vi "Generate skewed triangular waveform.vi"(4 "Duty cycle (%)":dbl, 5 "Offset":dbl, 6 "sampling info":cluster{"Fs":dbl, "#s":dbl}={"Fs"=1000.0, "#s"=1000.0} {"Fs" format="%.2p"}, 8 "error in (no error)":errorcluster, 9 "Phase":dbl, 10 "Amplitude":dbl, 11 "Frequency":dbl) -> (0 "error out":errorcluster, 3 "Waveform":waveform(dbl))   [LabVIEW 2012]
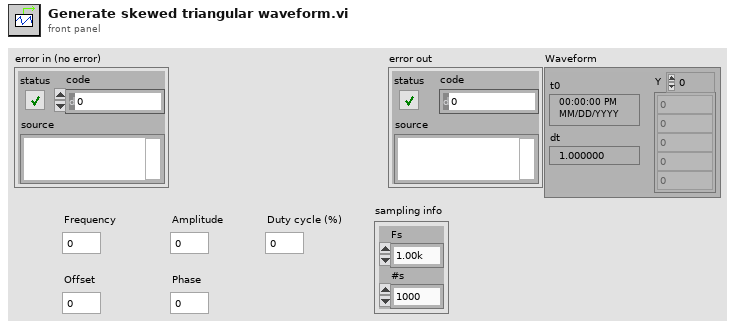
[diagram p1: front panel]
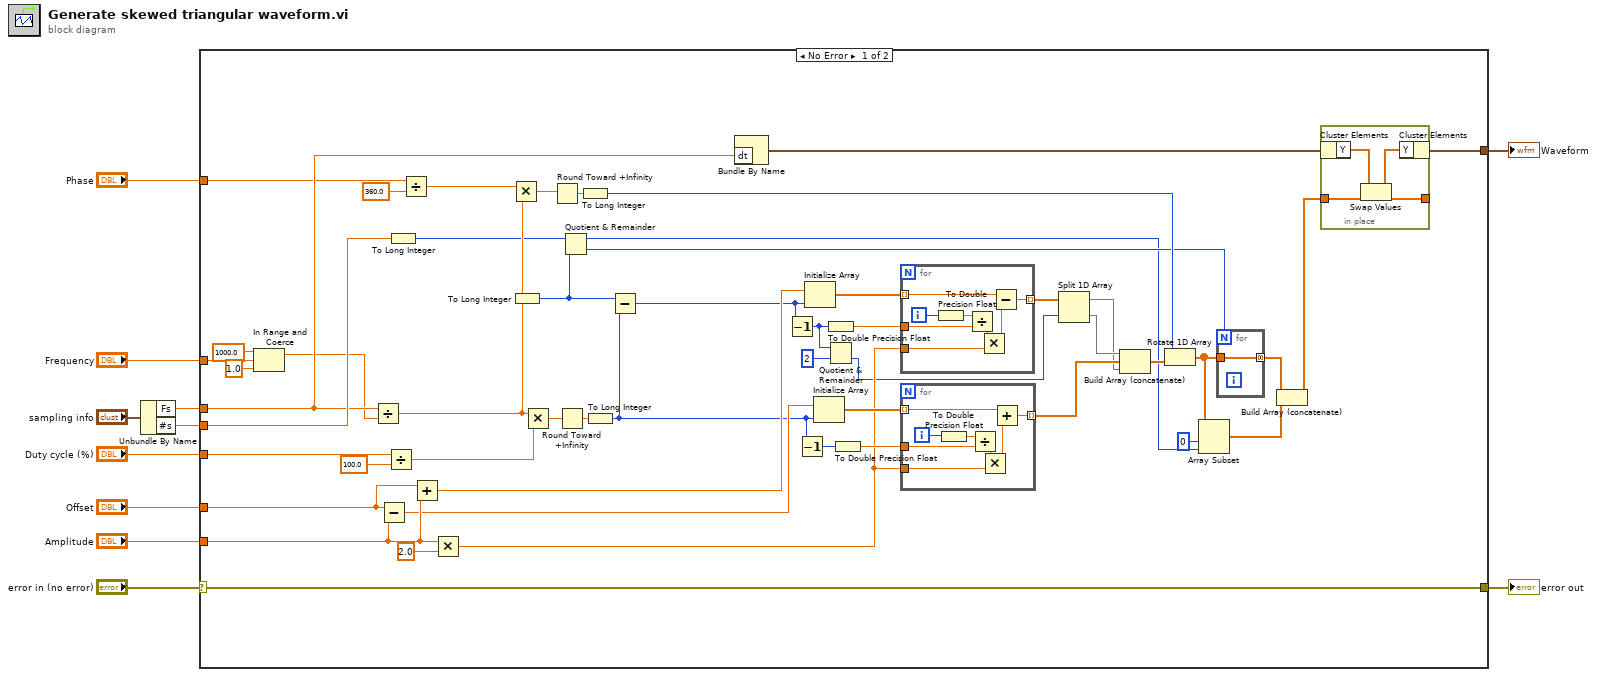
[diagram p0: block diagram]
diagram:
  n1 = Unbundle By Name("sampling info") -> ("Fs"=w4:dbl, "#s"=w7:dbl)
  n2 = case shown="No Error" "error in (no error)" {
    selector: "error in (no error)" -> [w56 w84]
    tunnel: [w56 w84] -> w10
    tunnel: [w55 _] -> w9
    tunnel: w7 -> [w62 _]
    tunnel: "Duty cycle (%)" -> [w61 _]
    tunnel: "Frequency" -> [w13 _]
    tunnel: w4 -> [w60 _]
    tunnel: "Amplitude" -> [w59 _]
    tunnel: "Offset" -> [w58 _]
    tunnel: "Phase" -> [w57 _]
    frame No Error {
      n3 = In Range and Coerce(upper limit=1000.0, x=w13, lower limit=1.0) -> (coerced(x)=w12:dbl)  [unwired: 1 out]
      n4 = Divide(x=w60, y=w12) -> (x/y=w32:dbl)
      n5 = Subtract(x=w58, y=w59) -> (x-y=w47:dbl)
      n6 = Divide(x=w61, y=100.0) -> (x/y=w53:dbl)
      n7 = To Long Integer(number=w62) -> (32bit integer=w29:i32)
      n8 = Divide(x=w57, y=360.0) -> (x/y=w31:dbl)
      n9 = Add(x=w58, y=w59) -> (x+y=w46:dbl)
      n10 = Multiply(x=w59, y=2.0) -> (x*y=w39:dbl)
      n11 = Multiply(x=w31, y=w32) -> (x*y=w35:dbl)
      n12 = To Long Integer(number=w32) -> (32bit integer=w30:i32)
      n13 = Multiply(x=w32, y=w53) -> (x*y=w50:dbl)
      n14 = Round Toward +Infinity(x=w35) -> (ceil(x): smallest int >= x=w36:dbl)
      n15 = Round Toward +Infinity(x=w50) -> (ceil(x): smallest int >= x=w54:dbl)
      n16 = Quotient & Remainder(x=w29, y=w30) -> (x-y*floor(x/y)=w26:i32, floor(x/y)=w28:i32)
      n17 = To Long Integer(number=w36) -> (32bit integer=w33:i32)
      n18 = To Long Integer(number=w54) -> (32bit integer=w45:i32)
      n19 = Subtract(x=w30, y=w45) -> (x-y=w43:i32)
      n20 = Bundle By Name("dt"=w60) -> (w51:waveform(dbl))  [unwired: 1 in]
      n21 = Decrement(x=w43) -> (x-1=w20:i32)
      n22 = Decrement(x=w45) -> (x-1=w42:i32)
      n23 = Initialize Array(w46, w43) -> (w48:dbl[])
      n24 = Initialize Array(w47, w45) -> (w49:dbl[])
      n25 = To Double Precision Float(number=w20) -> (double precision float=w40:dbl)
      n26 = Quotient & Remainder(x=w20, y=2) -> (floor(x/y)=w18:i32)  [unwired: 1 out]
      n27 = To Double Precision Float(number=w42) -> (double precision float=w41:dbl)
      n28 = for {
        tunnel: w48 -> [w65] mode=indexing
        tunnel: w40 -> [w69]
        tunnel: w39 -> [w68]
        tunnel: [w64] -> w21 mode=indexing
        i -> [w71]
        n29 = To Double Precision Float(number=w71) -> (double precision float=w70:dbl)
        n30 = Divide(x=w70, y=w69) -> (x/y=w67:dbl)
        n31 = Multiply(x=w67, y=w68) -> (x*y=w66:dbl)
        n32 = Subtract(x=w65, y=w66) -> (x-y=w64:dbl)
      }
      n33 = for {
        tunnel: w49 -> [w74] mode=indexing
        tunnel: w41 -> [w77]
        tunnel: w39 -> [w75]
        tunnel: [w72] -> w38 mode=indexing
        i -> [w79]
        n34 = To Double Precision Float(number=w79) -> (double precision float=w78:dbl)
        n35 = Divide(x=w78, y=w77) -> (x/y=w76:dbl)
        n36 = Multiply(x=w76, y=w75) -> (x*y=w73:dbl)
        n37 = Add(x=w74, y=w73) -> (x+y=w72:dbl)
      }
      n38 = Split 1D Array(array=w21, index=w18) -> (first subarray=w16:dbl[], second subarray=w17:dbl[])
      n39 = Build Array (concatenate)(w17, w38, w16) -> (w34:dbl[])
      n40 = Rotate 1D Array(1:w34, 2:w33) -> (0:w27:dbl[])
      n41 = Array Subset(array=w27, index=0, length=w26) -> (w24:dbl[])
      n42 = for {
        N: w28 -> [_]
        tunnel: w27 -> [w63]
        tunnel: [w63] -> w23 mode=concatenating
      }
      n43 = Build Array (concatenate)(w23, w24) -> (w22:dbl[])
      n44 = in-place {
        in-place-border: [w81] -> _
        in-place-border: w22 -> [w80]
        n45 = in-place-cluster #1(w51) -> ("Y"=w83:dbl[])
        n46 = Swap Values(12:w83, 14:w80) -> (1:w82:dbl[], 3:w81:dbl[])  [unwired: 1 in]
        n47 = in-place-cluster #1("Y"=w82) -> (w55:waveform(dbl))
      }
    }
    frame Error {
    }
  }
  "error out" <- w10
  "Waveform" <- w9
